vi "Drive Core.vi"() -> ()   [LabVIEW 2014]
uses:
  <vilib>/Rock Robotics/WPI/DriverStation/WPI_DriverStationRobotMode2.ctl
  <vilib>/Rock Robotics/Network Tables/SD Read Boolean.vi
  Begin/Global Variables.vi
  Begin/Global Constants.vi
  Begin/Global RefNums.vi
panel:
  in  "Min Correction":dbl=0.1
  in  "Reset Encoders":bool
  out "Counts FR":i32=881
  out "Counts FL":i32=731
  out "Counts BR":i32=531
  out "Counts BL":i32=477
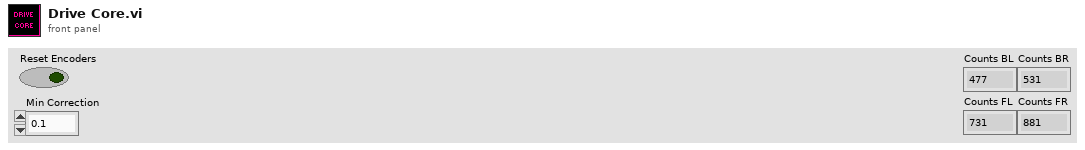
[diagram p1: front panel]
types:
  T1 = cluster{"Header P":dbl, "Header I":dbl, "Header D":dbl}
  T2 = typedef "WPI_DriverStationRobotMode2.ctl" = enum16{"Autonomous Disabled", "Autonomous Enabled", "Teleop Disabled", "Teleop Enabled", "Disconnected", "Finish", "Test Disabled", "Test Enabled", "Emergency Stopped"}
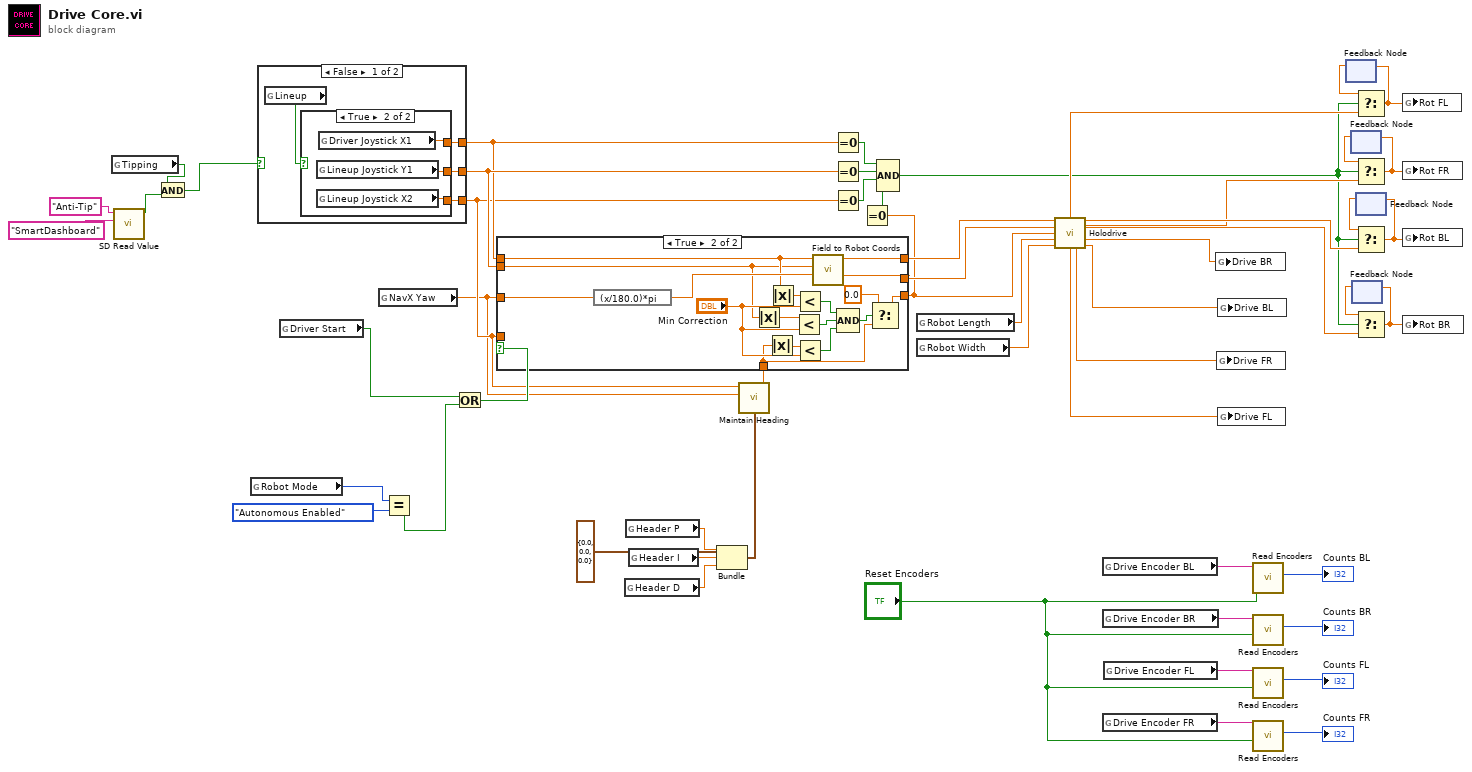
[diagram p0: block diagram]
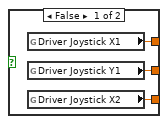
[diagram p2: hidden frame]
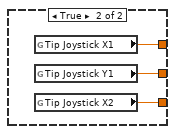
[diagram p3: hidden frame]
diagram:
  n1 = global read "Global Variables.vi" "Tipping"() -> (w14:bool)
  n2 = call-poly <vilib>:"SD Read Value.vi"("Table Prefix"="SmartDashboard", "Name"="Anti-Tip") -> ("Boolean"=w15:bool)  [unwired: 7 in, 2 out]
  n3 = And(x=w14, y=w15) -> (x .and. y?=w13:bool)
  n4 = global read "Global Variables.vi" "Robot Mode"() -> (w53:T2)
  n5 = case shown="False" w13 {
    tunnel: [w59 w66] -> w3
    tunnel: [w58 w67] -> w50
    tunnel: [w57 w68] -> w49
    frame False {
      n6 = global read "Global Variables.vi" "Lineup"() -> (w56:bool)
      n7 = case shown="True" w56 {
        tunnel: [w62 w63] -> w59
        tunnel: [w61 w64] -> w58
        tunnel: [w60 w65] -> w57
        frame False {
          n8 = global read "Global Variables.vi" "Driver Joystick X1"() -> (w60:dbl)
          n9 = global read "Global Variables.vi" "Driver Joystick Y1"() -> (w61:dbl)
          n10 = global read "Global Variables.vi" "Driver Joystick X2"() -> (w62:dbl)
        }
        frame True {
          n11 = global read "Global Variables.vi" "Lineup Joystick Y1"() -> (w64:dbl)
          n12 = global read "Global Variables.vi" "Lineup Joystick X2"() -> (w63:dbl)
          n13 = global read "Global Variables.vi" "Driver Joystick X1"() -> (w65:dbl)
        }
      }
    }
    frame True {
      n14 = global read "Global Variables.vi" "Tip Joystick X1"() -> (w68:dbl)
      n15 = global read "Global Variables.vi" "Tip Joystick Y1"() -> (w67:dbl)
      n16 = global read "Global Variables.vi" "Tip Joystick X2"() -> (w66:dbl)
    }
  }
  n17 = global read "Global Variables.vi" "Driver Start"() -> (w29:bool)
  n18 = global read "Global Variables.vi" "NavX Yaw"() -> (w2:dbl)
  n19 = Equal?(x=w53, y=WPI_DriverStationRobotMode2."Autonomous Enabled") -> (x = y?=w31:bool)
  n20 = Or(x=w29, y=w31) -> (x .or. y?=w30:bool)
  n21 = global read "Global Constants.vi" "Header D"() -> (w8:dbl)
  n22 = global read "Global Constants.vi" "Header P"() -> (w6:dbl)
  n23 = global read "Global Constants.vi" "Header I"() -> (w7:dbl)
  n24 = Bundle(cluster=T1 {"Header P"=0.0, "Header I"=0.0, "Header D"=0.0}, "Header P"=w6, "Header I"=w7, "Header D"=w8) -> (w4:T1)
  n25 = call "Maintain Heading.vi"("PID gains"=w4, "NavX Yaw"=w2, "Raw Driver Joystick X2"=w3) -> ("Driver Joystick X2"=w1:dbl)  [unwired: 8 in]
  n26 = case shown="True" w30 {
    tunnel: w49 -> [w71 w77]
    tunnel: w50 -> [w70 w74]
    tunnel: [w71 w85] -> w51
    tunnel: [w70 w88] -> w52
    tunnel: w3 -> [w69 _]
    tunnel: [w69 w84] -> w27
    tunnel: w2 -> [_ w86]
    tunnel: w1 -> [_ w72]
    frame False {
    }
    frame True {
      n27 = expression code="(x/180.0)*pi" ("degrees to radians")(w86) -> (w87:dbl)
      n28 = Absolute Value(x=w74) -> (abs(x)=w75:dbl)
      n29 = Absolute Value(x=w72) -> (abs(x)=w73:dbl)
      n30 = Absolute Value(x=w77) -> (abs(x)=w76:dbl)
      n31 = Less?(x=w75, y="Min Correction") -> (x < y?=w80:bool)
      n32 = Less?(x=w76, y="Min Correction") -> (x < y?=w81:bool)
      n33 = Less?(x=w73, y="Min Correction") -> (x < y?=w79:bool)
      n34 = call "Field to Robot Coords.vi"("gyro"=w87, "Joystick y"=w74, "Joystick x"=w77) -> ("robot y"=w88:dbl, "robot x"=w85:dbl)  [unwired: 7 in]
      n35 = Compound Arithmetic op=AND(w81, w80, w79) -> (w78:bool)
      n36 = Select(t=0.0, s=w78, f=w72) -> (s? t:f=w84:dbl)
    }
  }
  n37 = Equal To 0?(x=w49) -> (x = 0?=w32:bool)
  n38 = Equal To 0?(x=w50) -> (x = 0?=w33:bool)
  n39 = Equal To 0?(x=w3) -> (x = 0?=w34:bool)
  n40 = Equal To 0?(x=w27) -> (x = 0?=w28:bool)
  n41 = Compound Arithmetic op=AND(w32, w33, w34, w28) -> (w35:bool)
  n42 = global read "Global Constants.vi" "Robot Length"() -> (w54:dbl)
  n43 = global read "Global Constants.vi" "Robot Width"() -> (w55:dbl)
  n44 = call "Holodrive.vi"("Translation X"=w51, "Translation Y"=w52, "Angular"=w27, "Robot Length"=w54, "Robot Width"=w55) -> ("FL Rot"=w41:dbl, "FR Rot"=w38:dbl, "BL Rot"=w39:dbl, "BR Rot"=w40:dbl, "BR Drive"=w11:dbl, "FL Drive"=w9:dbl, "FR Drive"=w10:dbl, "BL Drive"=w12:dbl)  [unwired: 3 in]
  n45 = global read "Global RefNums.vi" "Drive Encoder BL"() -> (w26:string)
  n46 = global read "Global RefNums.vi" "Drive Encoder BR"() -> (w25:string)
  n47 = global read "Global RefNums.vi" "Drive Encoder FR"() -> (w23:string)
  n48 = global read "Global RefNums.vi" "Drive Encoder FL"() -> (w24:string)
  n49 = global write "Global Variables.vi" "Drive BR"(w11) -> ()
  n50 = global write "Global Variables.vi" "Drive FR"(w10) -> ()
  n51 = global write "Global Variables.vi" "Drive BL"(w12) -> ()
  n52 = global write "Global Variables.vi" "Drive FL"(w9) -> ()
  n53 = call "Read Encoders.vi"("Reset Encoders"="Reset Encoders", "Encoder"=w26) -> ("Counts"=→"Counts BL":i32)  [unwired: 9 in]
  n54 = call "Read Encoders.vi"("Reset Encoders"="Reset Encoders", "Encoder"=w25) -> ("Counts"=→"Counts BR":i32)  [unwired: 9 in]
  n55 = call "Read Encoders.vi"("Reset Encoders"="Reset Encoders", "Encoder"=w24) -> ("Counts"=→"Counts FL":i32)  [unwired: 9 in]
  n56 = call "Read Encoders.vi"("Reset Encoders"="Reset Encoders", "Encoder"=w23) -> ("Counts"=→"Counts FR":i32)  [unwired: 9 in]
  n57 = feedback #1() -> (w43:dbl)  [unwired: 1 in]
  n58 = feedback #2() -> (w37:dbl)  [unwired: 1 in]
  n59 = feedback #3() -> (w47:dbl)  [unwired: 1 in]
  n60 = Select(t=w43, s=w35, f=w41) -> (s? t:f=w42:dbl)
  n61 = feedback-in #1(w42) -> ()
  n62 = Select(t=w37, s=w35, f=w38) -> (s? t:f=w36:dbl)
  n63 = feedback-in #2(w36) -> ()
  n64 = feedback #4() -> (w45:dbl)  [unwired: 1 in]
  n65 = Select(t=w45, s=w35, f=w39) -> (s? t:f=w44:dbl)
  n66 = feedback-in #4(w44) -> ()
  n67 = Select(t=w47, s=w35, f=w40) -> (s? t:f=w46:dbl)
  n68 = feedback-in #3(w46) -> ()
  n69 = global write "Global Variables.vi" "Rot FL"(w42) -> ()
  n70 = global write "Global Variables.vi" "Rot FR"(w36) -> ()
  n71 = global write "Global Variables.vi" "Rot BL"(w44) -> ()
  n72 = global write "Global Variables.vi" "Rot BR"(w46) -> ()
